vi "Request_URL.vi"(8 "error in (no error)":errorcluster, 11 "LabVIEW Web Service Request":refnum<class "Web Request.lvclass">) -> (0 "error out":errorcluster, 2 "Request URL":string, 3 "LabVIEW Web Service Request out":refnum<class "Web Request.lvclass">)   [LabVIEW 2014]
doc: "Obtains the request URL"
uses:
  <vilib>/wsapi/Web Request.lvclass
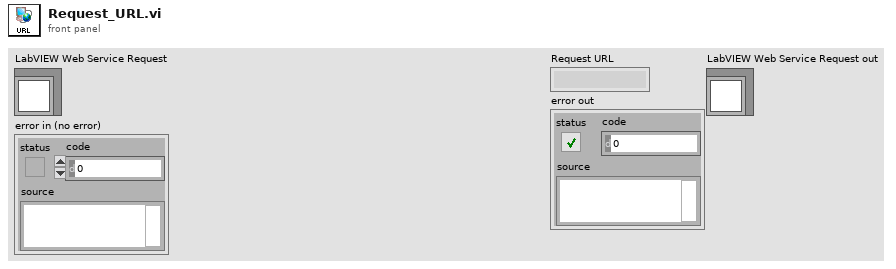
[diagram p1: front panel]
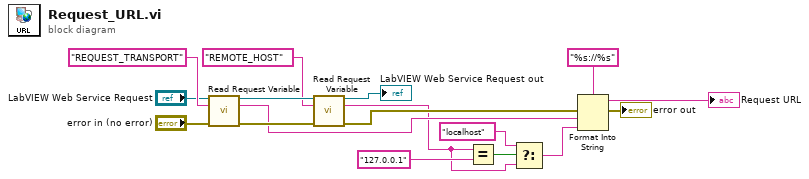
[diagram p0: block diagram]
diagram:
  n1 = call <vilib>:"Read Request Variable.vi"("LabVIEW Web Service Request"="LabVIEW Web Service Request", "variable name"="REQUEST_TRANSPORT", "error in (no error)"="error in (no error)") -> ("LabVIEW Web Service Request out"=w14:refnum<class "Web Request.lvclass">, "value"=w10:string, "error out"=w13:errorcluster)  [unwired: 10 in]
  n2 = call <vilib>:"Read Request Variable.vi"("LabVIEW Web Service Request"=w14, "variable name"="REMOTE_HOST", "error in (no error)"=w13) -> ("LabVIEW Web Service Request out"=→"LabVIEW Web Service Request out":refnum<class "Web Request.lvclass">, "value"=w2:string, "error out"=w9:errorcluster)  [unwired: 10 in]
  n3 = Equal?(x=w2, y="127.0.0.1") -> (x = y?=w5:bool)
  n4 = Select(t="localhost" ("y"), s=w5, f=w2) -> (s? t:f=w1:string)
  n5 = Format Into String(format string="%s://%s", error in=w9, w10, w1) -> (resulting string=→"Request URL":string, error out=→"error out":errorcluster)  [unwired: 1 in]
